vi "Load XML.vi"(7 "Program":string, 8 "error in (no error)":errorcluster caption="错误输入（无错误）", 9 "NAD":u8 format="%.0x", 10 "Send Data":refnum<vi>, 11 "XML File Path":path caption="XML文件路径") -> (1 "NAD":u8)   [LabVIEW 2018]
uses:
  Crl/LIN_DataType.ctl
  <vilib>/Utility/xml.llb/Read From XML File(string).vi
panel:
  # "ms"
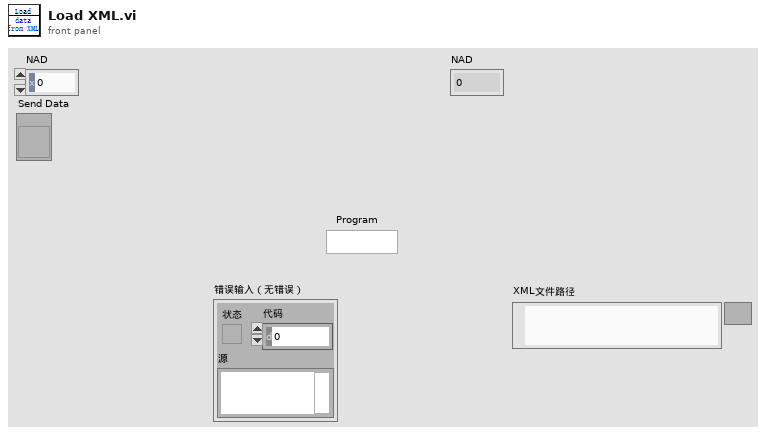
[diagram p1: front panel]
types:
  T1 = typedef "LIN_DataType.ctl" = cluster{"send?":bool, "payload":u8[], "Delays":u32, "Note":string, "mult?":bool, "Seq":i32}[]
  T2 = enum16{"open", "replace", "create", "open or create", "replace or create", "replace or create with confirmation"}
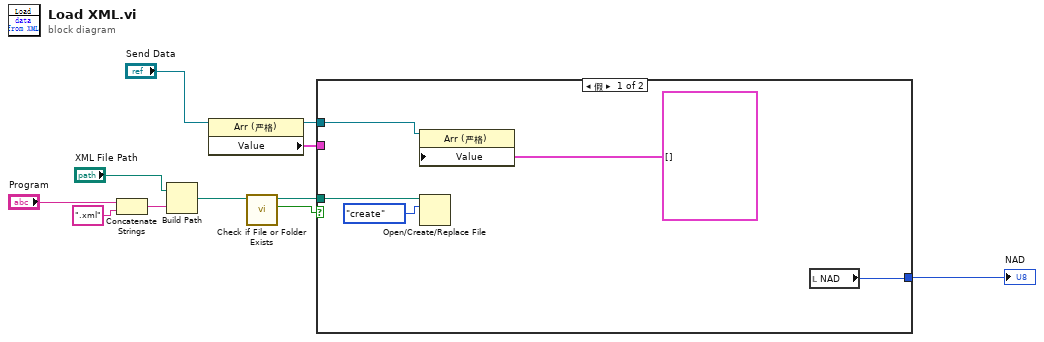
[diagram p0: block diagram]
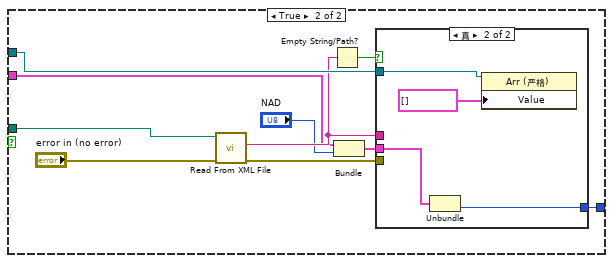
[diagram p2: hidden frame]
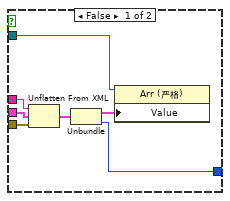
[diagram p3: hidden frame]
diagram:
  n1 = Concatenate Strings("Program", ".xml" ("字符串")) -> (w8:string)
  n2 = Build Path(base path="XML File Path", name or relative path=w8) -> (appended path=w7:path)
  n3 = property class="Arr (严格)"(reference="Send Data") -> (reference out=w4:refnum<vi>, "Value"=w3:T1)  [unwired: 1 in, 1 out]
  n4 = call <vilib>:"Check if File or Folder Exists.vi"("path"=w7) -> ("file or folder exists?"=w6:bool, "dup path"=w5:path)  [unwired: 8 in, 1 out]
  n5 = case shown="假" w6 {
    tunnel: w5 -> [w15 w25]
    tunnel: w4 -> [w14 w23]
    tunnel: w3 -> [_ w20]
    tunnel: [w12 w17] -> w2
    frame False {
      n6 = property class="Arr (严格)"(reference=w14, "Value"=T1 [] ("值")) -> ()  [unwired: 1 in, 2 out]
      n7 = Open/Create/Replace File(file path (use dialog)=w15, operation (0:open)=T2."create" ("操作(0:open)")) -> ()  [unwired: 4 in, 3 out]
      n8 = local read "NAD"() -> (w12:u8)
    }
    frame True {
      n9 = call-poly <vilib>:"Read From XML File.vi"("error in (no error)"="error in (no error)", "XML File Path"=w25) -> ("error out"=w26:errorcluster, "XML Elements"=w22:string)  [unwired: 7 in, 1 out]
      n10 = Empty String/Path?(string/path=w22) -> (empty?=w21:bool)
      n11 = Bundle("Value"=w20, "NAD"="NAD") -> (w18:cluster{"Value":T1, "NAD":u8})  [unwired: 1 in]
      n12 = case shown="真" w21 {
        tunnel: w26 -> [w33 _]
        tunnel: w23 -> [w32 w37]
        tunnel: w18 -> [w31 w35]
        tunnel: w22 -> [w30 _]
        tunnel: [w27 w34] -> w17
        frame False {
          n13 = Unflatten From XML(xml string=w30, type=w31, error in (no error)=w33) -> (value=w29:cluster{"Value":T1, "NAD":u8})  [unwired: 1 out]
          n14 = Unbundle(w29) -> ("Value"=w28:T1, "NAD"=w27:u8)
          n15 = property class="Arr (严格)"(reference=w32, "Value"=w28) -> ()  [unwired: 1 in, 2 out]
        }
        frame True {
          n16 = Unbundle(w35) -> ("NAD"=w34:u8)  [unwired: 1 out]
          n17 = property class="Arr (严格)"(reference=w37, "Value"=T1 [] ("值")) -> ()  [unwired: 1 in, 2 out]
        }
      }
    }
  }
  "NAD" <- w2
